vi "myRIO_BRig_RT_dataCurrent_laser2_triggered_ENL1.vi"() -> (2 "output_laser2_triggered_ENL1":i32)   [LabVIEW 2014]
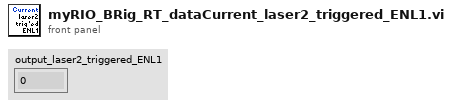
[diagram p1: front panel]
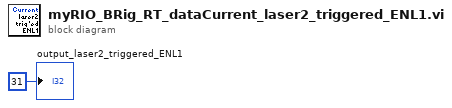
[diagram p0: block diagram]
diagram:
  "output_laser2_triggered_ENL1" <- 31 ("output_iBlock")
